vi "Main_18a.vi"() -> ()   [LabVIEW 2023]
uses:
  Problem-16/ENUM_Direction.ctl
  Cluster_Point.ctl
  <vilib>/Analysis/geometry.llb/Point in Polygon (Scalar).vi
  <vilib>/Analysis/geometry.llb/Point in Polygon Position.ctl
  <vilib>/Analysis/NI_AAL_Geometry.lvlib
panel:
  out "Array 4":T1[](array[typedef])
  out "Array 3":bool[](array[boolean])
  out "Numeric":i32
  out "Array 2":bool[][](array[boolean])
  out "Array":T3(array[cluster])
  out "Answer":i32
  in  "Puzzle":string="R 8 (#4cd962)\nU 10 (#6d5eb3)\nR 7 (#4cd960)\nU 3 (#5f8083)\nR 9 (#150a82)\nU 11 (#1af243)\nR 3 (#735892)\nU 8 (#14d253)\nR 4 (#4b5102)\nU 13 (#394313)\nL 4 (#6ca770)\nU 3 (#0f0fa3)\nR 8 (#6ca772)\nU 2 (#46a7e3)\nR 8 (#485eb2)\nU 9 (#1d0d03)\nL 4 (#32b972)\nU 4 (#379d31)\nL 5 (#61d940)\nU 8 (#43c751)\nL 4 (#61d942)\nD 8 (#30a311)\nL 6 (#0d4b12)\nD 4 (#3a14d3)\nL 8 (#523aa0)\nU 7 (#14af83)\nR 9 (#523aa2)\nU 8 (#381ea3)\nL 3 (#036240)\nD 5 (#5846b3)\nL 7 (#608040)\nU 5 (#2c73a3)\nL 8 (#4ef490)\nU 7 (#297a13)\nR 3 (#2eb380)\nU 4 (#34fb43)\nR 12 (#039a00)\nD 4 (#28a0b1)\nR 3 (#045110)\nU 3 (#54e2d1)\nR 8 (#045112)\nD 5 (#65ac21)\nR 4 (#13e780)\nD 13 (#5e2983)\nR 6 (#4e00b0)\nU 7 (#53ed43)\nR 9 (#150a80)\nU 5 (#5885c3)\nR 3 (#2bef82)\nD 2 (#314273)\nR 4 (#3389d2)\nD 10 (#2034f3)\nR 7 (#3d8692)\nD 3 (#2034f1)\nR 5 (#52fed2)\nD 7 (#06c7c3)\nR 7 (#1d7430)\nD 2 (#33d9c3)\nR 8 (#2fad00)\nD 11 (#3e9963)\nL 8 (#43c7e0)\nD 5 (#56c023)\nL 7 (#530960)\nD 6 (#41a7a1)\nL 12 (#777780)\nD 5 (#41a7a3)\nR 8 (#095620)\nD 8 (#436d61)\nR 8 (#3c5600)\nD 4 (#1352c1)\nR 9 (#3301c0)\nU 4 (#4be443)\nR 5 (#4c0b50)\nD 8 (#471793)\nL 3 (#59a050)\nD 4 (#240033)\nL 11 (#07a872)\nU 4 (#382b53)\nL 8 (#4eee22)\nD 11 (#382b51)\nR 6 (#4f1512)\nD 9 (#3324b3)\nR 6 (#322dc0)\nD 3 (#00d823)\nR 10 (#1d9902)\nD 10 (#03acb3)\nL 9 (#475d22)\nD 4 (#03acb1)\nL 5 (#332892)\nU 9 (#1bcc73)\nL 4 (#349a62)\nU 3 (#377f21)\nL 3 (#462992)\nD 2 (#377f23)\nL 6 (#1e5ff2)\nD 10 (#1bcc71)\nL 6 (#027302)\nU 4 (#5b1d33)\nL 3 (#632ee2)\nD 7 (#5b1d31)\nR 2 (#1b78e2)\nD 3 (#0699a3)\nR 10 (#53e842)\nD 4 (#69a413)\nR 5 (#049d22)\nD 4 (#3ff6e3)\nL 4 (#76e542)\nD 9 (#3c9453)\nR 4 (#73a9c2)\nD 8 (#1663a3)\nR 8 (#5bcbc2)\nU 7 (#219be1)\nR 8 (#356ba2)\nU 9 (#4e8441)\nL 8 (#356ba0)\nU 9 (#633221)\nR 11 (#4c38d2)\nD 3 (#574041)\nR 2 (#501392)\nD 9 (#6214c1)\nR 7 (#1e6b02)\nD 5 (#1d89a1)\nR 3 (#1d1762)\nU 9 (#1c29a1)\nR 11 (#1f9d32)\nU 5 (#5ac271)\nR 8 (#638532)\nU 9 (#464341)\nR 8 (#13b4c2)\nU 5 (#022b23)\nR 4 (#0c33f2)\nU 5 (#231bc1)\nR 4 (#25ab22)\nU 5 (#58ac91)\nL 6 (#5c1ee2)\nU 8 (#28d891)\nR 6 (#0ba3c2)\nU 4 (#0e3613)\nL 4 (#0fc262)\nU 6 (#3f2183)\nL 4 (#620da0)\nU 6 (#404db3)\nR 11 (#620da2)\nU 5 (#16fba3)\nR 3 (#11b8d2)\nU 13 (#022b21)\nR 3 (#0882e2)\nU 3 (#18ae53)\nL 4 (#3e3ed0)\nU 7 (#25b163)\nR 4 (#4820e2)\nU 5 (#263573)\nR 5 (#4820e0)\nD 5 (#369573)\nR 13 (#2d6140)\nD 6 (#805ff3)\nL 13 (#0f36f2)\nD 4 (#050f03)\nR 7 (#72de82)\nD 3 (#3eaba3)\nL 11 (#410332)\nD 8 (#4ee073)\nR 5 (#410330)\nD 4 (#2ee883)\nR 7 (#34c6a0)\nU 4 (#342b51)\nR 3 (#23e400)\nD 8 (#342b53)\nL 7 (#296ad0)\nD 4 (#30c0e3)\nL 5 (#440090)\nU 4 (#388373)\nL 3 (#5a32f0)\nD 7 (#107aa3)\nR 11 (#09a5b0)\nD 4 (#2533f3)\nL 4 (#6a2ef0)\nD 5 (#3edca3)\nR 6 (#097c20)\nD 6 (#0f8f33)\nR 6 (#4bd7a0)\nD 7 (#4e93b3)\nR 4 (#589750)\nU 12 (#2b30f3)\nR 3 (#253012)\nU 2 (#1546e3)\nR 6 (#3537a2)\nD 6 (#1546e1)\nR 3 (#4a0742)\nD 8 (#3195e3)\nR 5 (#361050)\nD 6 (#051b33)\nL 3 (#11ba70)\nD 5 (#570bb3)\nL 6 (#285582)\nD 8 (#1e7643)\nL 12 (#523062)\nD 3 (#1e7641)\nL 12 (#129462)\nD 5 (#54d8e3)\nR 4 (#3fa560)\nD 5 (#6298c3)\nR 5 (#3ddc40)\nD 4 (#6298c1)\nR 8 (#0f98a0)\nU 4 (#0589d3)\nR 4 (#587220)\nU 7 (#1dd5a3)\nR 6 (#0b0130)\nU 6 (#45e8a3)\nR 10 (#045be2)\nU 7 (#1634f3)\nR 4 (#045be0)\nU 10 (#3be3a3)\nL 4 (#0b0132)\nU 5 (#167553)\nR 3 (#5ac980)\nU 8 (#0f8223)\nR 2 (#2ea720)\nU 6 (#0a0621)\nR 5 (#261680)\nD 8 (#6357f1)\nR 4 (#44d220)\nD 7 (#0a2601)\nR 7 (#201880)\nD 10 (#45ca31)\nL 7 (#270940)\nD 9 (#3b1983)\nR 2 (#1ed210)\nD 4 (#4719c3)\nL 6 (#1ed212)\nD 7 (#025cc3)\nR 6 (#316870)\nD 4 (#38be43)\nR 3 (#5f1e40)\nU 2 (#2fc0d3)\nR 3 (#0a7682)\nU 6 (#535893)\nR 2 (#0a7680)\nU 7 (#1004f3)\nR 6 (#38e890)\nD 8 (#654883)\nR 2 (#40f0c0)\nD 5 (#479fb3)\nR 7 (#60c440)\nU 3 (#63c2f3)\nR 3 (#4fb462)\nU 11 (#555183)\nR 8 (#524372)\nU 12 (#1c6823)\nR 3 (#5121f2)\nU 4 (#4f3883)\nR 4 (#5121f0)\nU 5 (#4b79e3)\nR 8 (#7531b2)\nU 4 (#398fc3)\nR 4 (#123732)\nD 2 (#55f9c3)\nR 3 (#22ca72)\nD 7 (#354883)\nR 4 (#494ad2)\nD 5 (#0d0833)\nR 7 (#07dff0)\nD 8 (#6f0053)\nL 11 (#07dff2)\nD 5 (#07e113)\nR 4 (#0e36f0)\nD 7 (#3735d3)\nR 13 (#5b3010)\nD 5 (#599133)\nL 13 (#3f4980)\nD 3 (#0e5261)\nR 8 (#0d24f2)\nD 3 (#408901)\nR 9 (#0d24f0)\nD 3 (#3dea81)\nR 10 (#42eb80)\nD 3 (#05f363)\nL 4 (#2e2962)\nD 11 (#40af13)\nR 4 (#2e2960)\nD 3 (#462373)\nR 8 (#0bf740)\nD 5 (#4c1693)\nR 12 (#494ef0)\nD 3 (#4b6b23)\nR 7 (#49d6d2)\nD 7 (#2d52f1)\nR 6 (#4d4672)\nD 3 (#2d52f3)\nR 8 (#2062e2)\nD 9 (#1e1203)\nR 4 (#1ffb12)\nD 7 (#66af33)\nR 9 (#191132)\nD 3 (#099ef3)\nR 6 (#421ee2)\nD 9 (#1626a3)\nR 3 (#0e36f2)\nD 3 (#18c783)\nR 6 (#4ab2b0)\nU 3 (#133db3)\nR 8 (#17a8e0)\nU 4 (#2dffd3)\nR 4 (#477030)\nU 9 (#5b1803)\nR 8 (#2062d0)\nU 3 (#71aa23)\nR 5 (#0f44d0)\nU 11 (#2a6441)\nR 5 (#4924f0)\nU 5 (#775b71)\nR 6 (#1de5b0)\nD 5 (#775b73)\nR 5 (#37a850)\nU 5 (#451fe1)\nR 3 (#098290)\nU 6 (#1eb881)\nR 9 (#0f9ef0)\nU 6 (#7fc301)\nR 7 (#042e20)\nU 8 (#170a33)\nR 3 (#24bb30)\nU 8 (#457433)\nL 7 (#24bb32)\nU 4 (#4f50e3)\nL 11 (#6aacf0)\nU 4 (#3d7191)\nL 4 (#0b4730)\nU 7 (#055b71)\nL 5 (#64b562)\nU 7 (#089a21)\nL 9 (#2d3cc0)\nU 10 (#27ad91)\nL 3 (#3b5c50)\nU 7 (#1ba851)\nL 9 (#3780c2)\nU 2 (#4f9191)\nL 7 (#311852)\nU 10 (#177cf1)\nR 8 (#64b560)\nU 3 (#182521)\nL 13 (#0b4732)\nU 3 (#0f0961)\nL 2 (#134cf0)\nU 3 (#140cb1)\nR 11 (#5aaf10)\nU 4 (#33e313)\nR 4 (#29e480)\nU 3 (#2dca43)\nR 4 (#52c310)\nD 3 (#5ea8f3)\nR 5 (#52c312)\nD 8 (#1e7ad3)\nL 5 (#29e482)\nD 5 (#5235a3)\nR 6 (#060b50)\nD 7 (#679c93)\nR 5 (#555e20)\nU 2 (#044e33)\nR 6 (#401640)\nU 5 (#4aa1a3)\nR 7 (#3b9c10)\nU 4 (#39d943)\nR 5 (#464960)\nU 7 (#044853)\nR 5 (#3af3f0)\nU 4 (#7ccde3)\nR 7 (#1dcf90)\nD 8 (#1e18c1)\nR 4 (#271930)\nD 6 (#0d35b1)\nL 4 (#633060)\nD 6 (#5cd3e1)\nR 7 (#481540)\nU 3 (#1bcd01)\nR 5 (#653eb2)\nU 11 (#404f93)\nL 5 (#0f6c32)\nU 6 (#404f91)\nR 6 (#5db3f2)\nU 5 (#0a8781)\nR 5 (#478be0)\nU 4 (#6e5621)\nL 4 (#351470)\nU 11 (#258331)\nL 3 (#66acf0)\nU 11 (#2f2bb1)\nR 3 (#033da0)\nU 4 (#5b0833)\nR 4 (#07b590)\nU 4 (#4d3183)\nR 13 (#724800)\nD 5 (#3bff63)\nL 5 (#395930)\nD 4 (#6c5171)\nL 5 (#303540)\nD 9 (#4cb341)\nR 5 (#303542)\nD 3 (#2b3461)\nR 5 (#56b2d0)\nD 5 (#3ada31)\nR 9 (#22bba0)\nD 3 (#2ddf61)\nR 6 (#2e47d0)\nU 6 (#5a1571)\nR 4 (#2e47d2)\nU 7 (#295ff1)\nL 4 (#091df0)\nU 3 (#684971)\nR 7 (#2d4910)\nU 8 (#38f1b1)\nR 9 (#75c410)\nD 2 (#38f1b3)\nR 4 (#2d6850)\nD 5 (#508651)\nR 10 (#4e9ec0)\nD 4 (#108f83)\nR 5 (#0459c0)\nD 3 (#108f81)\nL 10 (#50d650)\nD 4 (#282921)\nL 5 (#02b5a0)\nD 6 (#526f81)\nR 4 (#2439c0)\nD 7 (#166291)\nR 6 (#22d310)\nD 4 (#2d01b1)\nR 6 (#5e2f00)\nU 10 (#5b2d11)\nR 7 (#16dcb0)\nD 10 (#258321)\nR 5 (#21dbb0)\nD 10 (#3cba21)\nL 8 (#41f790)\nD 6 (#17a9e1)\nL 10 (#74e962)\nD 5 (#3cdd11)\nR 9 (#3e1e72)\nD 7 (#5b9181)\nR 4 (#5ed7d0)\nD 9 (#35e751)\nR 6 (#5ed7d2)\nD 6 (#424671)\nR 6 (#6ce3f2)\nD 5 (#0d6011)\nL 8 (#180d90)\nD 3 (#193ea1)\nR 6 (#638c00)\nD 8 (#193ea3)\nL 6 (#19d7b0)\nD 7 (#053cd1)\nR 8 (#315290)\nD 5 (#1951f1)\nL 3 (#6638a2)\nD 7 (#38ed11)\nR 8 (#3151d2)\nD 5 (#001921)\nL 8 (#1d7cd0)\nD 3 (#358cf1)\nL 3 (#642860)\nD 5 (#3f88c1)\nL 6 (#15e540)\nD 4 (#2799f1)\nL 8 (#2fd3a0)\nD 6 (#7f5e11)\nL 5 (#451de0)\nU 3 (#7f5e13)\nL 2 (#0e2490)\nU 5 (#18b1b3)\nL 11 (#015f30)\nD 8 (#026403)\nL 5 (#590af2)\nU 6 (#2bfe93)\nL 3 (#67b4f0)\nD 5 (#47a6b3)\nL 2 (#67b4f2)\nD 7 (#335143)\nL 6 (#1288e2)\nD 4 (#271283)\nL 5 (#10bdb0)\nD 2 (#4af0d3)\nL 10 (#54cd20)\nD 2 (#19b203)\nL 2 (#658ad2)\nD 7 (#58e543)\nL 12 (#3b6340)\nD 4 (#1e1033)\nL 3 (#303090)\nD 9 (#5435b3)\nL 11 (#2aff50)\nD 6 (#34b5c1)\nL 6 (#3388a0)\nU 9 (#7abf31)\nL 2 (#4559a0)\nD 9 (#0338c1)\nL 6 (#35d160)\nU 7 (#285f41)\nL 8 (#3e2910)\nD 7 (#149d93)\nL 7 (#2ef080)\nD 6 (#4bd033)\nL 10 (#51a340)\nD 8 (#517d63)\nL 6 (#13c5e0)\nD 8 (#08b601)\nL 11 (#030490)\nD 3 (#03d191)\nR 5 (#31ebe0)\nD 11 (#3e81d1)\nL 5 (#1fade0)\nD 3 (#165c01)\nL 9 (#1fade2)\nU 3 (#314fb1)\nL 7 (#31ebe2)\nU 4 (#1b5941)\nL 7 (#5cfa40)\nU 6 (#03dcd1)\nR 14 (#265550)\nU 4 (#290791)\nL 6 (#1dbef2)\nU 8 (#6660f1)\nL 6 (#497772)\nU 4 (#50a851)\nL 6 (#220c12)\nU 10 (#144373)\nL 5 (#687912)\nD 10 (#144371)\nL 4 (#671b52)\nU 6 (#5dcee1)\nL 6 (#2a61d0)\nU 7 (#576f11)\nL 3 (#5a3610)\nD 7 (#321fa1)\nL 7 (#208a90)\nD 5 (#18fe01)\nL 4 (#57ff42)\nD 3 (#27de71)\nL 9 (#371e42)\nU 8 (#2bd741)\nL 8 (#1b2dc0)\nD 6 (#4fe5a1)\nL 6 (#677b60)\nD 4 (#0fdec1)\nL 5 (#1871b2)\nU 6 (#61e981)\nL 6 (#37a202)\nU 4 (#61e983)\nL 10 (#329572)\nD 4 (#0986e1)\nL 5 (#2596d2)\nD 10 (#5e58e3)\nR 5 (#638ea2)\nD 4 (#5ea813)\nL 5 (#1b7892)\nD 11 (#67e1f1)\nL 10 (#2ca1b2)\nD 11 (#1ca3b1)\nL 8 (#1441c2)\nD 3 (#492f91)\nL 6 (#11bc52)\nD 5 (#420851)\nR 6 (#691d42)\nD 4 (#0d9201)\nR 8 (#0709a2)\nD 3 (#0497e1)\nL 4 (#1d35e2)\nD 8 (#084121)\nL 10 (#5ec502)\nD 7 (#59fcd1)\nL 12 (#0a7642)\nU 3 (#135df1)\nL 5 (#2ea3f2)\nU 6 (#7dd381)\nL 9 (#0c7440)\nU 3 (#45f8c1)\nL 6 (#222852)\nU 4 (#07bbb1)\nR 3 (#465cf2)\nU 14 (#62da01)\nR 7 (#446b22)\nD 14 (#17ccd1)\nR 5 (#3229c0)\nU 5 (#0f4301)\nR 4 (#47d1b0)\nU 5 (#0f4303)\nR 4 (#32f4f0)\nU 7 (#272491)\nL 4 (#0c7442)\nU 5 (#18c2d1)\nL 4 (#1a39d2)\nU 3 (#5bf311)\nR 5 (#57a322)\nU 11 (#67f3a1)\nL 8 (#267492)\nD 3 (#3feac1)\nL 11 (#0241a2)\nD 9 (#0fe801)\nL 3 (#45e472)\nD 3 (#42f1f1)\nL 2 (#2aed70)\nD 6 (#1e6411)\nL 4 (#2aed72)\nD 4 (#42d321)\nR 4 (#2967c2)\nD 5 (#1dac71)\nL 6 (#11dd32)\nD 7 (#633151)\nL 10 (#58cb92)\nD 6 (#295ca1)\nL 6 (#23b052)\nU 3 (#409ad1)\nL 5 (#6f8bb2)\nU 7 (#3064f1)\nR 13 (#15ff42)\nU 3 (#583681)\nL 13 (#567282)\nU 7 (#441071)\nL 4 (#0cd092)\nU 7 (#4fa291)\nL 8 (#30aa42)\nU 8 (#144fe1)\nL 7 (#09fe32)\nU 11 (#4d0181)\nL 5 (#75f1c2)\nU 11 (#0f8961)\nL 8 (#09c082)\nU 3 (#115c71)\nL 5 (#362552)\nU 3 (#3e1851)\nL 4 (#282052)\nU 4 (#408121)\nL 11 (#2094c2)\nD 5 (#24bd73)\nL 2 (#2b2982)\nD 9 (#235531)\nL 12 (#4a8322)\nD 8 (#235533)\nL 12 (#167292)\nD 5 (#40be63)\nL 3 (#401f90)\nD 2 (#311e11)\nL 14 (#357b90)\nD 3 (#311e13)\nL 4 (#168410)\nU 10 (#2badc3)\nL 6 (#2c8df2)\nU 3 (#05c9c3)\nL 4 (#47bc12)\nU 9 (#518c73)\nL 7 (#2fd552)\nU 13 (#33c623)\nL 3 (#0eab22)\nU 11 (#2641d3)\nL 8 (#0a5380)\nU 8 (#3a1de3)\nL 6 (#407550)\nU 12 (#3a1de1)\nL 5 (#3b73b0)\nU 3 (#4624c3)\nL 8 (#026002)\nU 6 (#361063)\nL 7 (#5b5422)\nU 4 (#361061)\nL 2 (#3081f2)\nU 8 (#593d01)\nR 6 (#311f72)\nU 6 (#0a0c21)\nR 5 (#495672)\nU 5 (#778721)\nR 9 (#14a122)\nU 5 (#1cb2a1)\nR 3 (#0a3352)\nU 5 (#169e41)\nR 6 (#275ac0)\nU 4 (#4b0231)\nR 7 (#275ac2)\nU 6 (#2f8921)\nL 6 (#1a6e32)\nU 3 (#7a7171)\nL 4 (#2aa112)\nU 6 (#129dd1)\nL 4 (#321ca2)\nU 8 (#145083)\nR 4 (#144af2)\nU 4 (#3b48e3)\nL 7 (#0d5530)\nD 6 (#5d9413)\nL 5 (#0d5532)\nD 6 (#0c27e3)\nR 5 (#144af0)\nD 9 (#671013)\nL 5 (#0e28c2)\nU 6 (#12a133)\nL 5 (#378ef2)\nU 8 (#3eed61)\nL 5 (#6a5612)\nU 9 (#3edeb1)\nL 6 (#5dd080)\nU 7 (#025771)\nL 7 (#2ff460)\nU 4 (#617551)\nL 6 (#2ec2e2)\nD 4 (#40f7d1)\nL 3 (#5f0202)\nU 4 (#1075f1)\nL 6 (#2bf192)\nU 13 (#0580f3)"
  in  "Example":string="R 6 (#70c710)\nD 5 (#0dc571)\nL 2 (#5713f0)\nD 2 (#d2c081)\nR 2 (#59c680)\nD 2 (#411b91)\nL 5 (#8ceee2)\nU 2 (#caa173)\nL 1 (#1b58a2)\nU 2 (#caa171)\nR 2 (#7807d2)\nU 3 (#a77fa3)\nL 2 (#015232)\nU 2 (#7a21e3)"
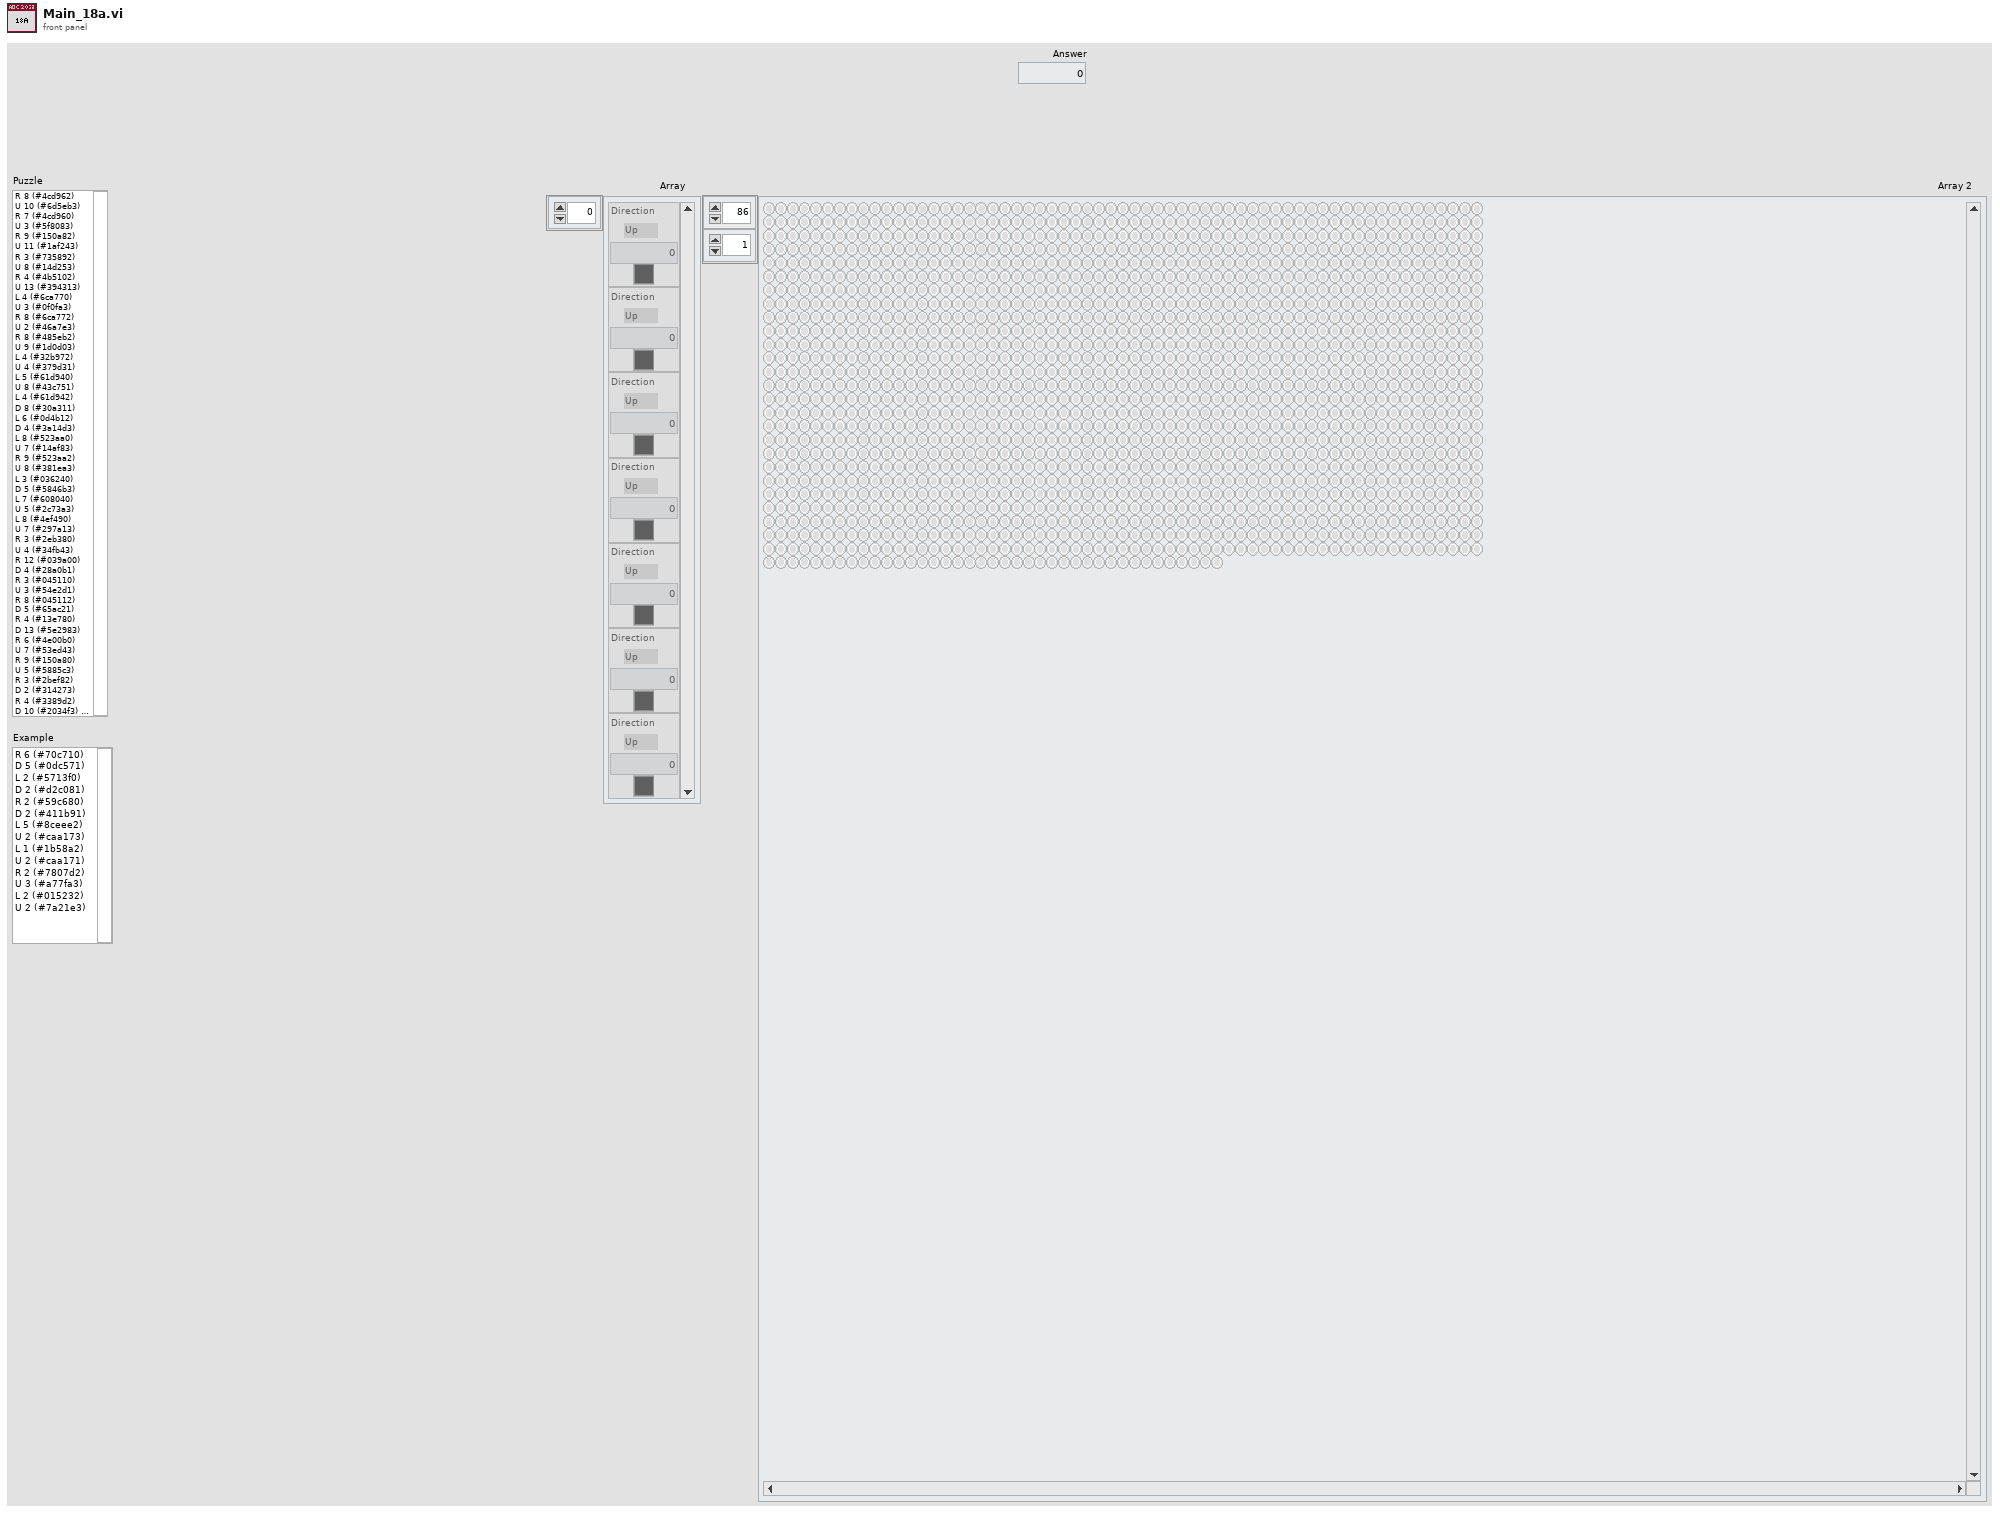
[diagram p1: front panel]
types:
  T1 = typedef "Cluster_Point.ctl" = cluster{"Row":i32, "Column":i32}
  T2 = typedef "ENUM_Direction.ctl" = enum16{"Up", "Left", "Down", "Right"}
  T3 = cluster{"Direction":T2, "Numeric":i32, "Color Box":u32}[]
  T4 = cluster{"Direction":T2, "count":i32, "Color":u32}
  T5 = typedef "NI_AAL_Geometry.lvlib/Point in Polygon Position.ctl" = u16
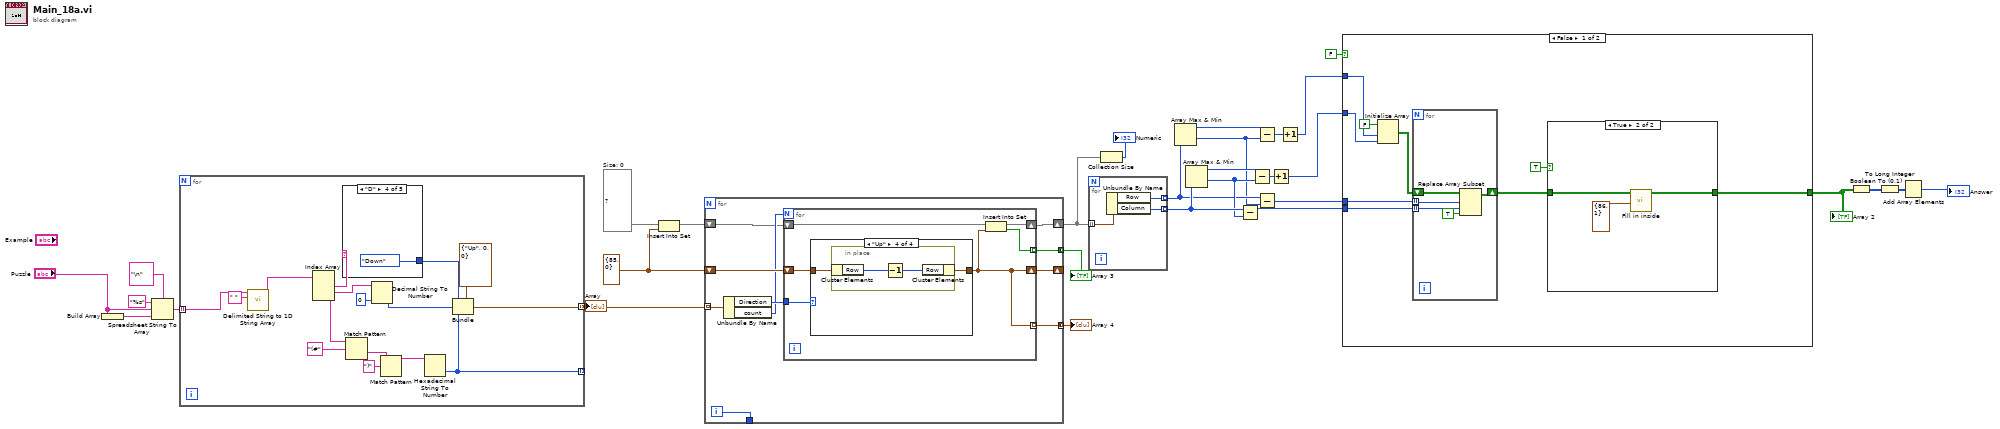
[diagram p0: block diagram]
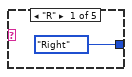
[diagram p2: hidden frame]
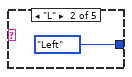
[diagram p3: hidden frame]
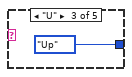
[diagram p4: hidden frame]
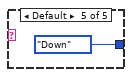
[diagram p5: hidden frame]
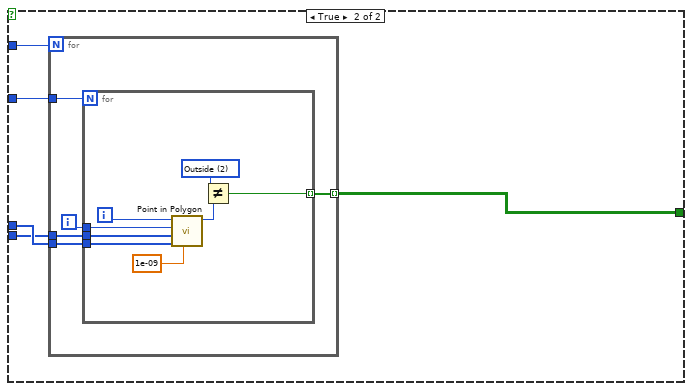
[diagram p7: hidden frame]
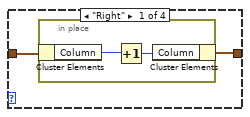
[diagram p8: hidden frame]
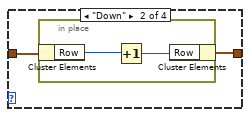
[diagram p9: hidden frame]
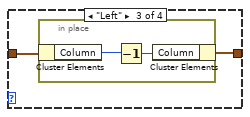
[diagram p10: hidden frame]
diagram:
  w24 = set{T1} {}  # Size: 0
  w25 = T1 {"Row"=85, "Column"=0} ("Point")
  n1 = Build Array("Puzzle") -> (w30:string[])
  n2 = Spreadsheet String To Array(delimiter (Tab)="\n", format string="%s", spreadsheet string="Puzzle", array type (2D Dbl)=w30) -> (array=w27:string[])
  n3 = for {
    tunnel: w27 -> [w46] mode=indexing
    tunnel: [w35] -> w26 mode=indexing
    tunnel: [w34] -> _ mode=indexing
    n4 = call <vilib>:"Delimited String to 1D String Array.vi"("delimiter"=" ", "delimited string"=w46) -> ("string array"=w44:string[])  [unwired: 9 in]
    n5 = Index Array(array=w44) -> (element #1=w43:string, element #2=w42:string, element #3=w40:string)  [unwired: 3 in]
    n6 = case shown="\"D\"" w43 {
      tunnel: [ENUM_Direction."Right" ("Direction") ENUM_Direction."Left" ("Direction") ENUM_Direction."Up" ("Direction") ENUM_Direction."Down" ("Direction") ENUM_Direction."Down" ("Direction")] -> w36
      frame "R" {
      }
      frame "L" {
      }
      frame "U" {
      }
      frame "D" {
      }
      frame Default {
      }
    }
    n7 = Match Pattern(string=w40, regular expression="(#") -> (after substring=w39:string)  [unwired: 1 in, 3 out]
    n8 = Decimal String To Number(string=w42, default (0L)=0 ("default (0 I32)")) -> (number=w32:i32)  [unwired: 1 in, 1 out]
    n9 = Match Pattern(string=w39, regular expression=")") -> (before substring=w37:string)  [unwired: 1 in, 3 out]
    n10 = Hexadecimal String To Number(string=w37) -> (number=w34:u32)  [unwired: 2 in, 1 out]
    n11 = Bundle(cluster=T4 {"Direction"=enum."Up", "count"=0, "Color"=0}, "Direction"=w36, "count"=w32, "Color"=w34) -> (w35:T4)
  }
  "Array" <- w26
  n12 = Insert Into Set(10:w25, 11:w24) -> (3:w23:set{T1})  [unwired: 1 out]
  n13 = for {
    tunnel: w26 -> [w61] mode=indexing
    shift-right: [w57] -> _
    shift-left: w25 -> [w60]
    shift-right: [w55] -> w7
    shift-left: w23 -> [w56]
    tunnel: [w54] -> w5 mode=concatenating
    tunnel: [w53] -> w4 mode=concatenating
    tunnel: [w52] -> _
    i -> [w52]
    n14 = Unbundle By Name(w61) -> ("Direction"=w59:T2, "count"=w58:i32)
    n15 = for {
      N: w58 -> [_]
      tunnel: w59 -> [w67]
      shift-right: [w64] -> w55
      shift-left: w56 -> [w65]
      shift-right: [w62] -> w57
      shift-left: w60 -> [w66]
      tunnel: [w63] -> w54 mode=indexing
      tunnel: [w62] -> w53 mode=indexing
      n16 = case shown="\"Up\"" w67 {
        tunnel: w66 -> [w69 w73 w77 w81]
        tunnel: [w68 w72 w76 w80] -> w62
        frame "Right" {
          n17 = in-place {
            n18 = in-place-cluster #1(w69) -> ("Column"=w71:i32)
            n19 = Increment(x=w71) -> (x+1=w70:i32)
            n20 = in-place-cluster #1("Column"=w70) -> (w68:T1)
          }
        }
        frame "Down" {
          n21 = in-place {
            n22 = in-place-cluster #2(w73) -> ("Row"=w75:i32)
            n23 = Increment(x=w75) -> (x+1=w74:i32)
            n24 = in-place-cluster #2("Row"=w74) -> (w72:T1)
          }
        }
        frame "Left" {
          n25 = in-place {
            n26 = in-place-cluster #3(w77) -> ("Column"=w79:i32)
            n27 = Decrement(x=w79) -> (x-1=w78:i32)
            n28 = in-place-cluster #3("Column"=w78) -> (w76:T1)
          }
        }
        frame "Up" {
          n29 = in-place {
            n30 = in-place-cluster #4(w81) -> ("Row"=w83:i32)
            n31 = Decrement(x=w83) -> (x-1=w82:i32)
            n32 = in-place-cluster #4("Row"=w82) -> (w80:T1)
          }
        }
      }
      n33 = Insert Into Set(10:w62, 11:w65) -> (2:w63:bool, 3:w64:set{T1})
    }
  }
  "Array 3" <- w5
  "Array 4" <- w4
  n34 = for {
    tunnel: w7 -> [w84] mode=indexing
    tunnel: [w86] -> w16 mode=indexing
    tunnel: [w85] -> w18 mode=indexing
    n35 = Unbundle By Name(w84) -> ("Row"=w86:i32, "Column"=w85:i32)
  }
  n36 = Collection Size(1:w7) -> (0:→"Numeric":i32)
  n37 = Array Max & Min(array=w16) -> (max value=w22:i32, min value=w15:i32)  [unwired: 2 out]
  n38 = Array Max & Min(array=w18) -> (max value=w21:i32, min value=w17:i32)  [unwired: 2 out]
  n39 = Subtract(x=w18, y=w17) -> (x-y=w3:i32[])
  n40 = Subtract(x=w21, y=w17) -> (x-y=w19:i32)
  n41 = Subtract(x=w22, y=w15) -> (x-y=w20:i32)
  n42 = Subtract(x=w16, y=w15) -> (x-y=w14:i32[])
  n43 = Increment(x=w19) -> (x+1=w12:i32)
  n44 = Increment(x=w20) -> (x+1=w13:i32)
  n45 = case shown="False" FALSE {
    tunnel: w14 -> [w90 w109]
    tunnel: w13 -> [w95 w108]
    tunnel: w12 -> [w94 w107]
    tunnel: [w89 w106] -> w11
    tunnel: w3 -> [w91 w105]
    frame False {
      n46 = Initialize Array(FALSE, w95, w94) -> (w92:bool[][])
      n47 = for {
        shift-right: [w103] -> w88
        shift-left: w92 -> [w104]
        tunnel: w91 -> [w100] mode=indexing
        tunnel: w90 -> [w101] mode=indexing
        n48 = Replace Array Subset(array=w104, new element=TRUE ("new element/subarray"), index (row)=w101, index (col)=w100) -> (w103:bool[][])
      }
      n49 = case shown="True" TRUE {
        tunnel: [w96 w99] -> w89
        tunnel: w88 -> [w96 w98]
        frame False {
        }
        frame True {
          n50 = call "Fill in inside.vi"("Starting Node"=T1 {"Row"=86, "Column"=1}, "Array in"=w98) -> ("Array out"=w99:bool[][])  [unwired: 9 in]
        }
      }
    }
    frame True {
      n51 = for {
        N: w108 -> [_]
        tunnel: w109 -> [w114]
        tunnel: w107 -> [w113]
        tunnel: [w111] -> w106 mode=indexing
        tunnel: w105 -> [w110]
        i -> [w112]
        n52 = for {
          N: w113 -> [_]
          tunnel: w114 -> [w116]
          tunnel: w112 -> [w121]
          tunnel: [w117] -> w111 mode=indexing
          tunnel: w110 -> [w115]
          i -> [w120]
          w119 = T5 2 items=["Inside", "On Boundary", "Outside"] ("position")
          n53 = call-poly <vilib>:"Point in Polygon.vi"("tolerance"=1e-09, "Polygon Y"=w116, "Polygon X"=w115, "y"=w121, "x"=w120) -> ("position"=w118:T5)  [unwired: 5 in, 1 out]
          n54 = Not Equal?(x=w119, y=w118) -> (x != y?=w117:bool)
        }
      }
    }
  }
  "Array 2" <- w11
  n55 = Boolean To (0,1)(Boolean=w11) -> (0, 1=w10:i16[][])
  n56 = To Long Integer(number=w10) -> (32bit integer=w9:i32[][])
  n57 = Add Array Elements(numeric array=w9) -> (sum=→"Answer":i32)
